vi "Build Custom Wfm.vi"(8 "error in":errorcluster, 10 "User Provided Name":string, 11 "Custom Wfm Config":T1={"File Path"="", "Sample Rate (Hz)"=10000000.0, "Read From"=0, "Pre Delay (s)"=0.0, "Post Delay (s)"=0.0, "Scale"=1.0} {"Scale" min=0.0 format="%#_6p"; "Read From" min=0; "Pre Delay (s)" min=0.0 format="%#_6p"; "Sample Rate (Hz)" min=0.0 format="%#_6p"; "Post Delay (s)" min=0.0 format="%#_6p"}) -> (0 "error out":errorcluster, 1 "Actual Duration (s)":dbl format="%#_6p", 2 "Actual Sample Size":i32, 3 "Waveform":waveform(dbl)(graph))   [LabVIEW 2025, in "TDMS Waveform Creator UI.lvlib"]
uses:
  TDMS Waveform Creator UI.lvlib
  <vilib>/Utility/file.llb/Read Delimited Spreadsheet (string).vi
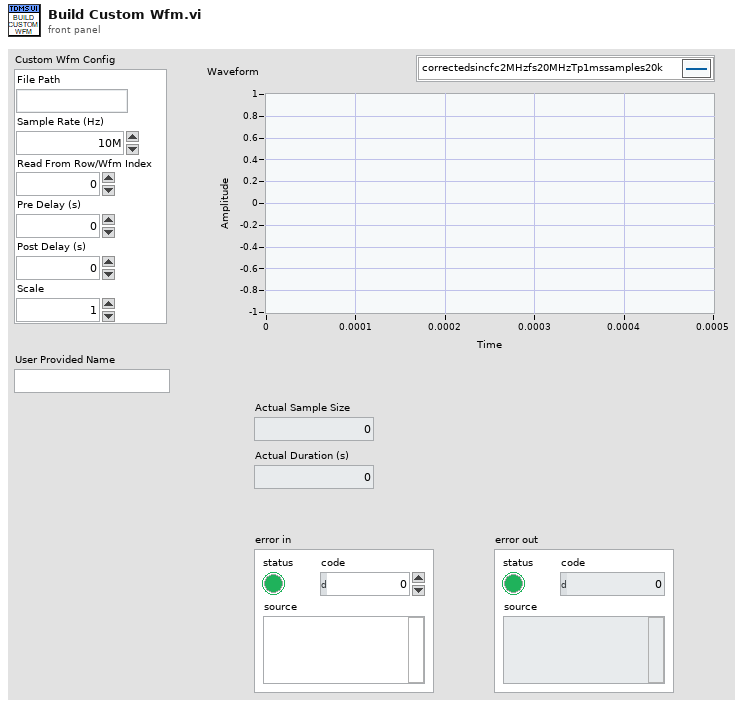
[diagram p1: front panel]
types:
  T1 = cluster{"File Path":string, "Sample Rate (Hz)":dbl, "Read From":i32, "Pre Delay (s)":dbl, "Post Delay (s)":dbl, "Scale":dbl}
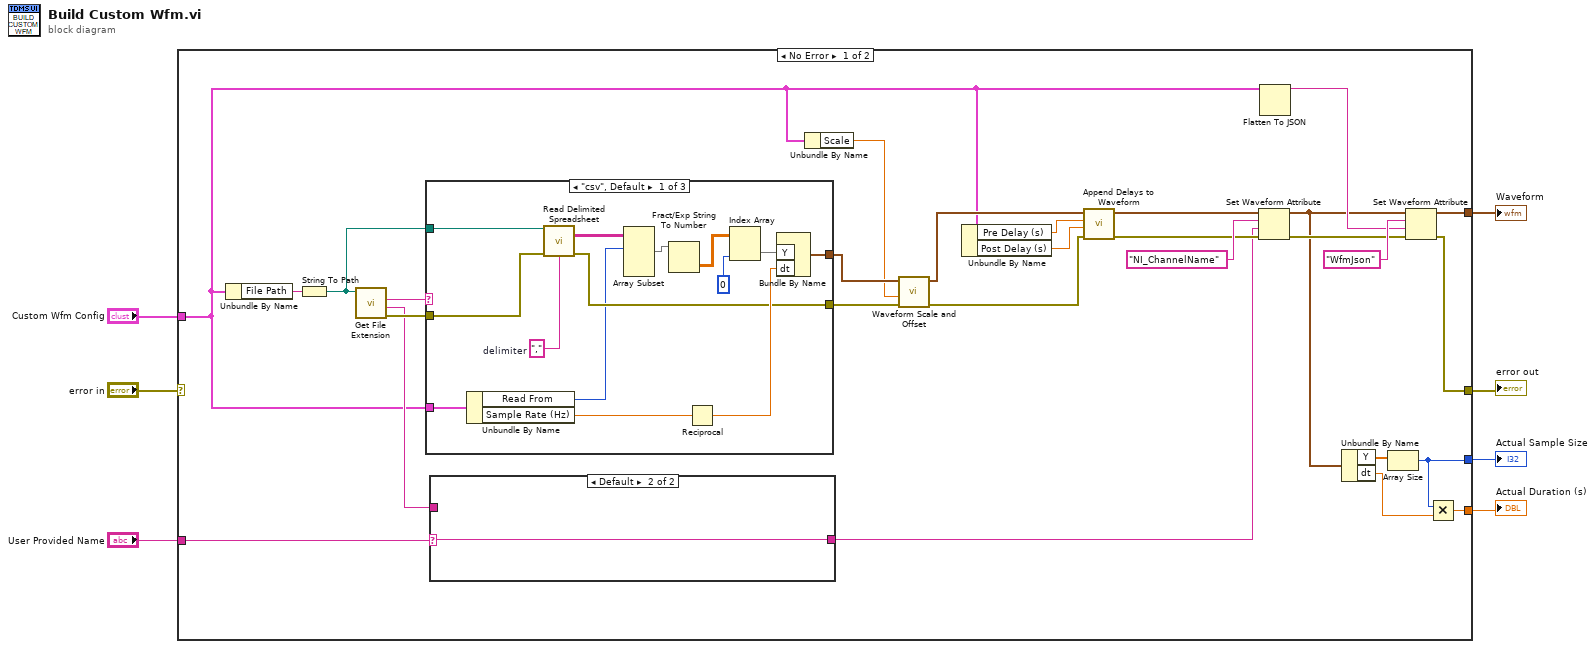
[diagram p0: block diagram]
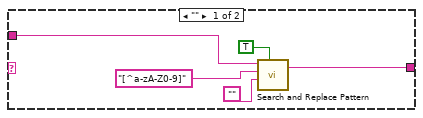
[diagram p2: hidden frame]
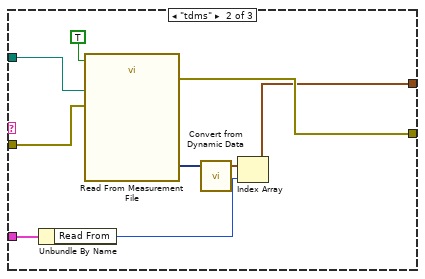
[diagram p3: hidden frame]
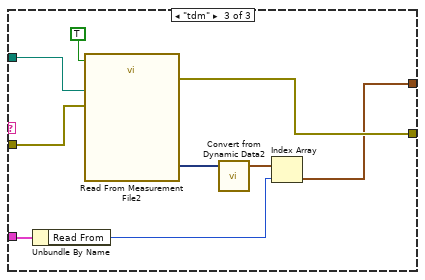
[diagram p4: hidden frame]
diagram:
  n1 = case shown="No Error" "error in" {
    selector: "error in" -> [_ w74]
    tunnel: "Custom Wfm Config" -> [w9 _]
    tunnel: [w31 _] -> w6
    tunnel: [w30 w74] -> w4
    tunnel: [w21 _] -> w3
    tunnel: [w20 _] -> w2
    tunnel: "User Provided Name" -> [w19 _]
    frame No Error {
      n2 = Unbundle By Name(w9) -> ("File Path"=w18:string)
      n3 = String To Path(string=w18) -> (path=w14:path)
      n4 = call <vilib>:"Get File Extension.vi"("file"=w14) -> ("error out"=w16:errorcluster, "filename without extension"=w15:string, "lowercase file extension"=w25:string)  [unwired: 6 in, 2 out]
      n5 = case shown="\"csv\", Default" w25 {
        tunnel: w14 -> [w54 w64 w73]
        tunnel: [w47 w60 w69] -> w11
        tunnel: [w46 w63 w72] -> w13
        tunnel: w9 -> [w44 w58 w67]
        tunnel: w16 -> [w42 w56 w65]
        frame "csv", Default {
          w55 = ","  # delimiter
          n6 = Unbundle By Name(w44) -> ("Read From"=w43:i32, "Sample Rate (Hz)"=w45:dbl)
          n7 = call-poly <vilib>:"Read Delimited Spreadsheet.vi"("file path (dialog if empty)"=w54, "error in (no error)"=w42, "delimiter (\\t)"=w55) -> ("all rows"=w51:string[][], "error out"=w46:errorcluster)  [unwired: 7 in, 4 out]
          n8 = Array Subset(array=w51, index (row)=w43) -> (w50:string[][])  [unwired: 3 in]
          n9 = Fract/Exp String To Number(string=w50) -> (number=w49:dbl[][])  [unwired: 3 in, 1 out]
          n10 = Reciprocal(x=w45) -> (1/x=w52:dbl)
          n11 = Index Array(array=w49, index (col)=0) -> (element=w48:dbl[])  [unwired: 1 in]
          n12 = Bundle By Name("Y"=w48, "dt"=w52) -> (w47:waveform(dbl))  [unwired: 1 in]
        }
        frame "tdms" {
          n13 = Unbundle By Name(w58) -> ("Read From"=w57:i32)
          n14 = call "Read From Measurement File"("error in (no error)"=w56, "Filename"=w64, "Reset"=TRUE) -> ("error out"=w63:errorcluster, "Signals"=w62:dynamicdata)  [unwired: 3 in, 4 out]
          n15 = call "Convert from Dynamic Data"("Dynamic Data Type"=w62) -> ("Array of Waveform"=w61:waveform(dbl)[])  [unwired: 3 in]
          n16 = Index Array(array=w61, index=w57) -> (element=w60:waveform(dbl))
        }
        frame "tdm" {
          n17 = Unbundle By Name(w67) -> ("Read From"=w66:i32)
          n18 = call "Read From Measurement File2"("error in (no error)"=w65, "Filename"=w73, "Reset"=TRUE) -> ("error out"=w72:errorcluster, "Signals"=w71:dynamicdata)  [unwired: 3 in, 4 out]
          n19 = call "Convert from Dynamic Data2"("Dynamic Data Type"=w71) -> ("Array of Waveform"=w70:waveform(dbl)[])  [unwired: 3 in]
          n20 = Index Array(array=w70, index=w66) -> (element=w69:waveform(dbl))
        }
      }
      n21 = case shown="Default" w19 {
        selector: w19 -> [_ w41]
        tunnel: [w37 w41] -> w17
        tunnel: w15 -> [w36 _]
        frame "" {
          n22 = call <vilib>:"Search and Replace Pattern.vi"("string"=w36, "regular expression (\"\")"="[^a-zA-Z0-9]" ("regular expression"), "replace string (\"\")"="" ("replace string (\"\")"), "replace all? (F)"=TRUE) -> ("result string"=w37:string)  [unwired: 1 in, 1 out]
        }
        frame Default {
        }
      }
      n23 = Unbundle By Name(w9) -> ("Scale"=w8:dbl)
      n24 = call <vilib>:"Waveform Scale and Offset.vi"("error in (no error)"=w13, "scale"=w8, "waveform in"=w11) -> ("error out"=w12:errorcluster, "waveform out"=w10:waveform(dbl))  [unwired: 7 in]
      n25 = Unbundle By Name(w9) -> ("Pre Delay (s)"=w27:dbl, "Post Delay (s)"=w26:dbl)
      n26 = call "Append Delays to Waveform.vi"("error in (no error)"=w12, "Post Delay (s)"=w26, "Pre Delay (s)"=w27, "Input Waveform"=w10) -> ("error out"=w28:errorcluster, "Output Waveform"=w29:waveform(dbl))  [unwired: 6 in]
      n27 = Set Waveform Attribute(4:w28, 5:w17, 6:"NI_ChannelName" ("name"), 7:w29) -> (0:w34:errorcluster, 3:w22:waveform(dbl))  [unwired: 1 out]
      n28 = Flatten To JSON(anything=w9) -> (JSON string=w32:string)  [unwired: 2 in, 1 out]
      n29 = Unbundle By Name(w22) -> ("Y"=w23:dbl[], "dt"=w24:dbl)
      n30 = Array Size(array=w23) -> (size(s)=w21:i32)
      n31 = Set Waveform Attribute(4:w34, 5:w32, 6:"WfmJson" ("name"), 7:w22) -> (0:w30:errorcluster, 3:w31:waveform(dbl))  [unwired: 1 out]
      n32 = Multiply(x=w21, y=w24) -> (x*y=w20:dbl)
    }
    frame Error {
    }
  }
  "Actual Duration (s)" <- w2
  "Actual Sample Size" <- w3
  "Waveform" <- w6
  "error out" <- w4
